vi "Stepper -- V5.vi"() -> ()   [LabVIEW 2019]
doc: "Use this template to build a producer/consumer design pattern with events to produce queue items. Use this design pattern instead of the User Interface Event Handler pattern for user interfaces when you want to execute code asynchronously in response to an event without slowing the user interface responsiveness."
uses:
  stepper motor state.ctl
  cursor range mode.ctl
  motor type.ctl
  stepper graphics action.ctl
  stepper driver action.ctl
  stepper progress monitor message.ctl
  talkto async routine action.ctl
  stepper graphics internal state.ctl
  stepper graphics internal event.ctl
  slider action.ctl
  stepper driver -- BLM.vi
  publisher action.ctl
panel:
  in  "Tab Control":enum32{"main", "init&stuff", "ignore", "calc"}(tab)
  in  "cur step":dbl(slide) scale=-5725.0..5322.0 scale format="%#.0f"
  in  "set step !":dbl(slide)=882.0 min=0.0 max=16000.0 step=1.0 scale=-5725.0..5322.0
  in  "set angle!":dbl(slide)=21.577803928668402 scale=-110.0..110.0
  in  "Stop!":bool
  in  "Go!":bool
  in  "check!":bool
  in  "stepper state":T1=enum."stopped"
  in  "XY Graph":cluster{dbl[], dbl[]}[](graph)=[{[-0.27897570766599245, -0.2006667370930823, -0.12235776652017213, -0.044048795947261965, 0.034260174625648177, 0.11256914519855832, 0.19087811577146852, 0.2691870863443786, 0.3474960569172888, 0.425805027490199, 0.5041139980631091, 0.5824229686360193, 0.6607319392089295, 0.7390409097818396, 0.8173498803547496, 0.89565885092766, 0.97396782150057, 1.0522767920734801, 1.1305857626463904, 1.2088947332193005], [-0.11032930042494946, -0.07935967223548995, -0.04839004404603046, -0.01742041585657096, 0.013549212332888541, 0.04451884052234803, 0.07548846871180753, 0.10645809690126704, 0.13742772509072654, 0.16839735328018604, 0.19936698146964552, 0.23033660965910505, 0.26130623784856455, 0.292275866038024, 0.3232454942274835, 0.3542151224169431, 0.38518475060640256, 0.41615437879586203, 0.4471240069853215, 0.478093635174781]}, {[-0.29926451263811893, -0.23626145734588336, -0.1732584020536478, -0.11025534676141222, -0.047252291469176644, 0.015750763823058955, 0.0787538191152945, 0.14175687440753004, 0.20475992969976564, 0.26776298499200124, 0.33076604028423684, 0.3937690955764723, 0.4567721508687079, 0.5197752061609435, 0.582778261453179, 0.6457813167454146, 0.7087843720376502, 0.7717874273298858, 0.8347904826221214, 0.897793537914357], [-0.020994081915366267, -0.01657427519634179, -0.01215446847731731, -0.007734661758292832, -0.0033148550392683544, 0.0011049516797561228, 0.005524758398780603, 0.00994456511780508, 0.014364371836829558, 0.018784178555854035, 0.023203985274878512, 0.02762379199390299, 0.032043598712927474, 0.03646340543195195, 0.04088321215097643, 0.045303018870000905, 0.04972282558902538, 0.05414263230804986, 0.05856243902707434, 0.06298224574609881]}, {[1.0, 0.9980267284282716, 0.9921147013144779, 0.9822872507286887, 0.9685831611286311, 0.9510565162951535, 0.9297764858882513, 0.9048270524660195, 0.8763066800438636, 0.8443279255020151, 0.8090169943749475, 0.7705132427757891, 0.7289686274214116, 0.6845471059286886, 0.6374239897486896, 0.587785252292473, 0.5358267949789965, 0.48175367410171516, 0.42577929156507266, 0.36812455268467786, 0.30901699437494745, 0.24868988716485474, 0.18738131458572452, 0.12533323356430426, 0.0627905195293133, -1.6081428723391245e-16, -0.0627905195293134, -0.12533323356430437, -0.18738131458572482, -0.24868988716485485, -0.30901699437494756, -0.368124552684678, -0.4257792915650727, -0.48175367410171543, -0.5358267949789969, -0.587785252292473, -0.6374239897486897, -0.6845471059286887, -0.7289686274214117, -0.7705132427757894, -0.8090169943749473, -0.8443279255020151, -0.8763066800438636, -0.9048270524660196, -0.9297764858882515, -0.9510565162951536, -0.9685831611286311, -0.9822872507286887, -0.9921147013144779, -0.9980267284282716, -1.0, -0.9980267284282716, -0.9921147013144779, -0.9822872507286886, -0.9685831611286311, -0.9510565162951535, -0.9297764858882512, -0.9048270524660195, -0.8763066800438635, -0.844327925502015, -0.8090169943749472, -0.770513242775789, -0.7289686274214116, -0.6845471059286886, -0.6374239897486895, -0.5877852522924732, -0.5358267949789963, -0.48175367410171527, -0.42577929156507216, -0.3681245526846778, -0.30901699437494756, -0.24868988716485443, -0.18738131458572463, -0.12533323356430373, -0.06279051952931321, -1.836909530733566e-16, 0.06279051952931372, 0.12533323356430423, 0.18738131458572513, 0.24868988716485493, 0.30901699437494723, 0.36812455268467825, 0.4257792915650726, 0.4817536741017157, 0.5358267949789968, 0.5877852522924737, 0.63742398974869, 0.6845471059286886, 0.7289686274214119, 0.7705132427757894, 0.8090169943749478, 0.8443279255020153, 0.8763066800438636, 0.9048270524660197, 0.9297764858882515, 0.9510565162951538, 0.9685831611286312, 0.9822872507286887, 0.9921147013144779, 0.9980267284282716], [0.0, 0.06279051952931337, 0.12533323356430426, 0.18738131458572463, 0.2486898871648548, 0.3090169943749474, 0.368124552684678, 0.4257792915650727, 0.4817536741017153, 0.5358267949789967, 0.5877852522924731, 0.6374239897486897, 0.6845471059286887, 0.7289686274214116, 0.7705132427757893, 0.8090169943749475, 0.8443279255020151, 0.8763066800438637, 0.9048270524660196, 0.9297764858882515, 0.9510565162951535, 0.9685831611286311, 0.9822872507286887, 0.9921147013144779, 0.9980267284282716, 1.0, 0.9980267284282716, 0.9921147013144778, 0.9822872507286886, 0.9685831611286311, 0.9510565162951535, 0.9297764858882513, 0.9048270524660195, 0.8763066800438635, 0.844327925502015, 0.8090169943749475, 0.7705132427757893, 0.7289686274214114, 0.6845471059286885, 0.6374239897486895, 0.5877852522924732, 0.5358267949789967, 0.4817536741017152, 0.4257792915650725, 0.36812455268467775, 0.3090169943749471, 0.24868988716485482, 0.18738131458572457, 0.1253332335643041, 0.06279051952931314, -3.216285744678249e-16, -0.06279051952931335, -0.12533323356430429, -0.18738131458572477, -0.24868988716485502, -0.30901699437494773, -0.3681245526846783, -0.42577929156507266, -0.4817536741017154, -0.5358267949789968, -0.5877852522924734, -0.63742398974869, -0.6845471059286887, -0.7289686274214116, -0.7705132427757894, -0.8090169943749473, -0.8443279255020153, -0.8763066800438636, -0.9048270524660198, -0.9297764858882515, -0.9510565162951535, -0.9685831611286312, -0.9822872507286887, -0.9921147013144779, -0.9980267284282716, -1.0, -0.9980267284282716, -0.9921147013144779, -0.9822872507286886, -0.9685831611286311, -0.9510565162951536, -0.9297764858882512, -0.9048270524660196, -0.8763066800438634, -0.844327925502015, -0.809016994374947, -0.770513242775789, -0.7289686274214116, -0.6845471059286883, -0.6374239897486896, -0.5877852522924726, -0.5358267949789963, -0.4817536741017153, -0.4257792915650722, -0.36812455268467786, -0.3090169943749468, -0.2486898871648545, -0.18738131458572468, -0.1253332335643038, -0.06279051952931326]}, {[0.1, 0.09980267284282716, 0.0992114701314478, 0.09822872507286887, 0.09685831611286312, 0.09510565162951537, 0.09297764858882515, 0.09048270524660196, 0.08763066800438636, 0.08443279255020152, 0.08090169943749474, 0.07705132427757892, 0.07289686274214115, 0.06845471059286887, 0.06374239897486897, 0.05877852522924731, 0.05358267949789966, 0.04817536741017152, 0.042577929156507266, 0.03681245526846779, 0.03090169943749475, 0.024868988716485477, 0.018738131458572452, 0.012533323356430426, 0.00627905195293133, -1.6081428723391246e-17, -0.0062790519529313405, -0.012533323356430436, -0.018738131458572484, -0.024868988716485487, -0.030901699437494757, -0.0368124552684678, -0.04257792915650727, -0.048175367410171546, -0.05358267949789969, -0.05877852522924731, -0.06374239897486897, -0.06845471059286888, -0.07289686274214117, -0.07705132427757895, -0.08090169943749474, -0.08443279255020152, -0.08763066800438636, -0.09048270524660197, -0.09297764858882515, -0.09510565162951537, -0.09685831611286312, -0.09822872507286888, -0.0992114701314478, -0.09980267284282716, -0.1, -0.09980267284282716, -0.0992114701314478, -0.09822872507286887, -0.09685831611286311, -0.09510565162951536, -0.09297764858882514, -0.09048270524660196, -0.08763066800438636, -0.0844327925502015, -0.08090169943749473, -0.07705132427757891, -0.07289686274214116, -0.06845471059286887, -0.06374239897486896, -0.05877852522924733, -0.05358267949789963, -0.04817536741017153, -0.04257792915650722, -0.036812455268467784, -0.03090169943749476, -0.024868988716485445, -0.018738131458572463, -0.012533323356430372, -0.0062790519529313206, -1.836909530733566e-17, 0.006279051952931373, 0.012533323356430424, 0.018738131458572515, 0.024868988716485498, 0.030901699437494726, 0.03681245526846783, 0.042577929156507266, 0.048175367410171574, 0.053582679497899674, 0.05877852522924737, 0.063742398974869, 0.06845471059286887, 0.07289686274214119, 0.07705132427757894, 0.08090169943749478, 0.08443279255020153, 0.08763066800438636, 0.09048270524660197, 0.09297764858882515, 0.09510565162951538, 0.09685831611286312, 0.09822872507286887, 0.0992114701314478, 0.09980267284282716], [0.0, 0.006279051952931338, 0.012533323356430426, 0.018738131458572466, 0.02486898871648548, 0.030901699437494743, 0.0368124552684678, 0.04257792915650727, 0.04817536741017153, 0.05358267949789967, 0.058778525229247314, 0.06374239897486898, 0.06845471059286887, 0.07289686274214116, 0.07705132427757894, 0.08090169943749476, 0.08443279255020152, 0.08763066800438638, 0.09048270524660196, 0.09297764858882515, 0.09510565162951536, 0.09685831611286312, 0.09822872507286888, 0.0992114701314478, 0.09980267284282716, 0.1, 0.09980267284282716, 0.0992114701314478, 0.09822872507286887, 0.09685831611286312, 0.09510565162951536, 0.09297764858882515, 0.09048270524660196, 0.08763066800438636, 0.0844327925502015, 0.08090169943749476, 0.07705132427757892, 0.07289686274214115, 0.06845471059286885, 0.06374239897486896, 0.05877852522924732, 0.05358267949789967, 0.048175367410171525, 0.04257792915650725, 0.03681245526846778, 0.030901699437494712, 0.024868988716485484, 0.01873813145857246, 0.01253332335643041, 0.0062790519529313145, -3.216285744678249e-17, -0.0062790519529313344, -0.012533323356430431, -0.018738131458572477, -0.0248689887164855, -0.030901699437494774, -0.03681245526846783, -0.04257792915650727, -0.04817536741017154, -0.05358267949789968, -0.05877852522924734, -0.06374239897486901, -0.06845471059286887, -0.07289686274214116, -0.07705132427757894, -0.08090169943749474, -0.08443279255020153, -0.08763066800438636, -0.09048270524660199, -0.09297764858882515, -0.09510565162951536, -0.09685831611286312, -0.09822872507286888, -0.0992114701314478, -0.09980267284282716, -0.1, -0.09980267284282716, -0.0992114701314478, -0.09822872507286887, -0.09685831611286311, -0.09510565162951537, -0.09297764858882514, -0.09048270524660196, -0.08763066800438633, -0.0844327925502015, -0.0809016994374947, -0.07705132427757891, -0.07289686274214116, -0.06845471059286884, -0.06374239897486897, -0.058778525229247265, -0.05358267949789964, -0.04817536741017153, -0.042577929156507224, -0.036812455268467784, -0.03090169943749468, -0.024868988716485452, -0.01873813145857247, -0.012533323356430379, -0.006279051952931327]}, {[-1.7, -1.7, -1.7, -1.7, -1.7, -1.7, -1.7, -1.7, -1.7, -1.7, -1.7, -1.7, -1.7, -1.7, -1.7, -1.7, -1.7, -1.7, -1.7, -1.7, -1.7, -1.6105263157894736, -1.5210526315789474, -1.431578947368421, -1.3421052631578947, -1.2526315789473683, -1.163157894736842, -1.0736842105263158, -0.9842105263157894, -0.894736842105263, -0.8052631578947368, -0.7157894736842105, -0.6263157894736842, -0.5368421052631578, -0.44736842105263164, -0.35789473684210527, -0.2684210526315789, -0.17894736842105252, -0.08947368421052615, 0.0, 0.0, 0.08947368421052632, 0.17894736842105263, 0.26842105263157895, 0.35789473684210527, 0.4473684210526316, 0.5368421052631579, 0.6263157894736842, 0.7157894736842105, 0.8052631578947369, 0.8947368421052632, 0.9842105263157894, 1.0736842105263158, 1.1631578947368422, 1.2526315789473683, 1.3421052631578947, 1.431578947368421, 1.5210526315789474, 1.6105263157894738, 1.7, 1.7, 1.7, 1.7, 1.7, 1.7, 1.7, 1.7, 1.7, 1.7, 1.7, 1.7, 1.7, 1.7, 1.7, 1.7, 1.7, 1.7, 1.7, 1.7, 1.7], [1.9, 1.7210526315789472, 1.5421052631578946, 1.3631578947368421, 1.1842105263157894, 1.0052631578947366, 0.8263157894736841, 0.6473684210526316, 0.46842105263157885, 0.2894736842105261, 0.11052631578947358, -0.06842105263157894, -0.24736842105263168, -0.4263157894736844, -0.6052631578947367, -0.7842105263157895, -0.9631578947368422, -1.142105263157895, -1.3210526315789477, -1.5, -1.5, -1.5257894736842106, -1.551578947368421, -1.5773684210526315, -1.6031578947368421, -1.6289473684210527, -1.654736842105263, -1.6805263157894736, -1.7063157894736842, -1.7321052631578948, -1.7578947368421052, -1.7836842105263158, -1.8094736842105263, -1.8352631578947367, -1.8610526315789473, -1.8868421052631579, -1.9126315789473685, -1.938421052631579, -1.9642105263157894, -1.99, -1.9900000000000002, -1.9642105263157896, -1.9384210526315793, -1.9126315789473687, -1.886842105263158, -1.8610526315789475, -1.8352631578947372, -1.8094736842105266, -1.783684210526316, -1.7578947368421054, -1.732105263157895, -1.7063157894736845, -1.6805263157894739, -1.6547368421052635, -1.628947368421053, -1.6031578947368423, -1.5773684210526318, -1.5515789473684212, -1.5257894736842108, -1.5000000000000002, -1.5, -1.3210526315789473, -1.1421052631578947, -0.9631578947368421, -0.7842105263157895, -0.6052631578947368, -0.4263157894736842, -0.24736842105263168, -0.06842105263157894, 0.1105263157894738, 0.2894736842105263, 0.46842105263157885, 0.6473684210526316, 0.8263157894736843, 1.0052631578947366, 1.1842105263157894, 1.3631578947368421, 1.5421052631578949, 1.7210526315789476, 1.9]}, {[-0.3420201433256687, -0.3492205673956828, -0.3564209914656969, -0.3636214155357109, -0.370821839605725, -0.3780222636757391, -0.3852226877457532, -0.3924231118157673, -0.3996235358857813, -0.4068239599557954, -0.4140243840258095, -0.4212248080958236, -0.4284252321658376, -0.4356256562358517, -0.4428260803058658, -0.4500265043758799, -0.45722692844589397, -0.46442735251590805, -0.47162777658592214, -0.4788282006559362], [0.9396926207859084, 0.9594756233287697, 0.9792586258716309, 0.9990416284144921, 1.0188246309573534, 1.0386076335002146, 1.0583906360430757, 1.078173638585937, 1.0979566411287982, 1.1177396436716593, 1.1375226462145207, 1.1573056487573818, 1.177088651300243, 1.1968716538431043, 1.2166546563859655, 1.2364376589288266, 1.256220661471688, 1.2760036640145493, 1.2957866665574105, 1.3155696691002716]}, {[-0.3420201433256687, -0.3492205673956828, -0.3564209914656969, -0.3636214155357109, -0.370821839605725, -0.3780222636757391, -0.3852226877457532, -0.3924231118157673, -0.3996235358857813, -0.4068239599557954, -0.4140243840258095, -0.4212248080958236, -0.4284252321658376, -0.4356256562358517, -0.4428260803058658, -0.4500265043758799, -0.45722692844589397, -0.46442735251590805, -0.47162777658592214, -0.4788282006559362], [-0.9396926207859084, -0.9594756233287697, -0.9792586258716309, -0.9990416284144921, -1.0188246309573534, -1.0386076335002146, -1.0583906360430757, -1.078173638585937, -1.0979566411287982, -1.1177396436716593, -1.1375226462145207, -1.1573056487573818, -1.177088651300243, -1.1968716538431043, -1.2166546563859655, -1.2364376589288266, -1.256220661471688, -1.2760036640145493, -1.2957866665574105, -1.3155696691002716]}, {[-0.4788282006559362, -0.42797342694834783, -0.37648774886137176, -0.3244470648918203, -0.27192809170796073, -0.2190082510563231, -0.16576555562910145, -0.11227849406040255, -0.058625915220879475, -0.004886911981313146, 0.04885929538350151, 0.10253347597868427, 0.15605650508885563, 0.2093494808211934, 0.2623338404200143, 0.31493147608141087, 0.36706485009721057, 0.41865710915852133, 0.4696321976503571, 0.5199149697703286, 0.5694313003061202, 0.6181081939084433, 0.6658738926983852, 0.7126579820505197, 0.7583914943958358, 0.8030070108914645, 0.8464387608073247, 0.8886227184831744, 0.9294966977131381, 0.9690004434185695, 1.0070757204741114, 1.043666399556007, 1.0787185398861048, 1.1121804687495853, 1.1440028576691799, 1.1741387951235935, 1.20254385570293, 1.2291761655991726, 1.2539964643351778, 1.276968162641182, 1.2980573963935023, 1.3172330765359155, 1.3344669349101257, 1.349733565927754, 1.3630104640224243, 1.3742780568267294, 1.383519734025174, 1.390721871840555, 1.3958738531176882, 1.3989680829748696, 1.4, 1.3989680829748696, 1.3958738531176882, 1.390721871840555, 1.383519734025174, 1.3742780568267294, 1.3630104640224243, 1.3497335659277543, 1.3344669349101257, 1.3172330765359157, 1.2980573963935025, 1.2769681626411822, 1.253996464335178, 1.2291761655991726, 1.2025438557029302, 1.1741387951235938, 1.1440028576691799, 1.1121804687495855, 1.0787185398861048, 1.0436663995560072, 1.0070757204741119, 0.9690004434185695, 0.9294966977131384, 0.888622718483175, 0.8464387608073248, 0.8030070108914648, 0.7583914943958362, 0.7126579820505199, 0.6658738926983856, 0.6181081939084433, 0.5694313003061205, 0.5199149697703291, 0.4696321976503571, 0.41865710915852167, 0.36706485009721057, 0.3149314760814112, 0.2623338404200149, 0.2093494808211934, 0.15605650508885596, 0.1025334759786849, 0.04885929538350151, -0.004886911981312835, -0.05862591522087885, -0.11227849406040225, -0.16576555562910084, -0.2190082510563231, -0.27192809170796045, -0.3244470648918197, -0.37648774886137176, -0.4279734269483475], [-1.3155696691002716, -1.332981149838994, -1.3484275935167214, -1.361886229493155, -1.373337217488868, -1.3827636768331928, -1.3901517113491517, -1.395490429838746, -1.3987719621384016, -1.3999914707209065, -1.3991471578267338, -1.3962402681142412, -1.391275086824835, -1.3842589334658082, -1.3752021510201642, -1.3641180906993293, -1.351023092261236, -1.3359364599227874, -1.3188804339022153, -1.299880157633279, -1.2789636406996412, -1.2561617175440598, -1.2315080020132632, -1.205038837805521, -1.176793244893958, -1.1468128620045883, -1.1151418852338748, -1.0818270028962915, -1.0469173266979446, -1.010464319337707, -0.9725217186425963, -0.9331454583492336, -0.8923935856481656, -0.8503261756126013, -0.8070052426377105, -0.762494649021038, -0.7168600108188002, -0.6701686011168495, -0.6224892508588987, -0.573892247378202, -0.5244492307822769, -0.47423308834340794, -0.42331784705062225, -0.3717785644815325, -0.31969121815491813, -0.2671325935271628, -0.21418017079765359, -0.16091201069001346, -0.10740663937754624, -0.05374293272252798, 0.0, 0.05374293272252768, 0.10740663937754594, 0.16091201069001315, 0.21418017079765295, 0.2671325935271628, 0.31969121815491786, 0.3717785644815319, 0.42331784705062225, 0.47423308834340766, 0.5244492307822763, 0.5738922473782017, 0.6224892508588982, 0.6701686011168495, 0.7168600108187999, 0.7624946490210375, 0.8070052426377105, 0.850326175612601, 0.8923935856481656, 0.9331454583492333, 0.9725217186425958, 1.010464319337707, 1.0469173266979444, 1.081827002896291, 1.1151418852338746, 1.1468128620045883, 1.1767932448939575, 1.205038837805521, 1.2315080020132627, 1.2561617175440598, 1.278963640699641, 1.2998801576332786, 1.3188804339022153, 1.3359364599227874, 1.351023092261236, 1.364118090699329, 1.375202151020164, 1.3842589334658082, 1.391275086824835, 1.3962402681142412, 1.3991471578267338, 1.3999914707209065, 1.3987719621384016, 1.395490429838746, 1.3901517113491517, 1.3827636768331928, 1.3733372174888683, 1.3618862294931553, 1.3484275935167214, 1.3329811498389943]}]
  in  "motor selector":T2=enum."BLM"
  in  "Instrument Address":refnum<visa-resource-name>="ASRL21::INSTR"
  in  "set speed!":bool
  in  "speed":dbl=0.4 format="%_2f"
  in  "sync to":bool
  in  "syncto":dbl format="%_2f"
  in  "cursor mode":T3
  in  "response message":cluster{"step (fdeg)":dbl}={"step (fdeg)"=310.3875004849805}
  out "progress monitor VI":refnum<vi>
  out "cur angle":dbl(slide)=4.0128541685525505 scale=-110.0..110.0 scale format="%#.0f"
  in  "angle aux":dbl(slide)=110.0 scale=-90.0..90.0 scale format="%#.0f"
  in  "step aux":dbl(slide)=5322.333333333334 scale=-4721.0..4318.0 scale format="%#.0f"
  in  "dir":u16(ring)
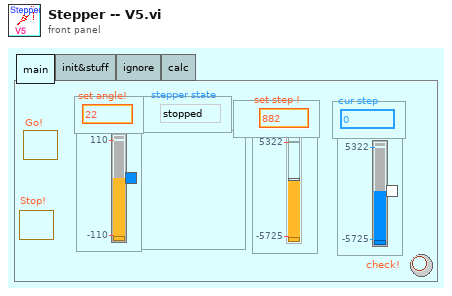
[diagram p1: front panel]
types:
  T1 = typedef "stepper motor state.ctl" = enum16{"moving", "stopped"}
  T2 = typedef "motor type.ctl" = enum16{"IMS", "arduino C&A", "BLM", "--"}
  T3 = typedef "cursor range mode.ctl" = enum16{"change angle", "lock", "extend"}
  T4 = typedef "stepper graphics action.ctl" = enum16{"--update circle", "set step slider moves", "cursor moves", "current step changed", "init", "void", "--draw current line", "--draw set line", "--move current step slider", "--move set step slider", "--draw limit lines", "check", "--move set angle slider", "--move current angle slider", "set angle slider moves", "--move center cursor", "set set step", "set current step", "read", "--move limit-cursors", "cursor release", "current step moves"}
  T5 = typedef "stepper driver action.ctl" = enum16{"go", "void", "stop", "check", "init", "sync", "set", "set speed", "--check status", "--check value", "--handshake"}
  T6 = typedef "stepper graphics internal event.ctl" = enum16{"set slider moves", "update scale", "exit", "current positon changed", "stop", "go", "set speed", "set to zero", "sync", "check"}
  T7 = typedef "stepper graphics internal state.ctl" = cluster{"set pos slider":refnum<vi>, "cur angle slider":refnum<vi>, "XY Graph":refnum<vi>, "set angle":dbl, "current angle":dbl, "set angle slider":refnum<vi>, "current pos... slider":refnum<vi>, "current pos":dbl, "set pos":dbl}
  T8 = typedef "talkto async routine action.ctl" = enum16{"stop", "check"}
  T9 = typedef "stepper progress monitor message.ctl" = cluster{"current position":dbl, "stepper motor state OUT":T1}
  T10 = typedef "publisher action.ctl" = enum16{"set", "get", "init", "check"}
  T11 = typedef "slider action.ctl" = enum16{"check", "copy range -- keep value", "set from value", "set from ratio", "set from slider", "read using other slider", "set lower limit", "set upper limit", "set lower from slider", "set upper from slider", "copy range -- keep ratio", "set using other slider -- no check"}
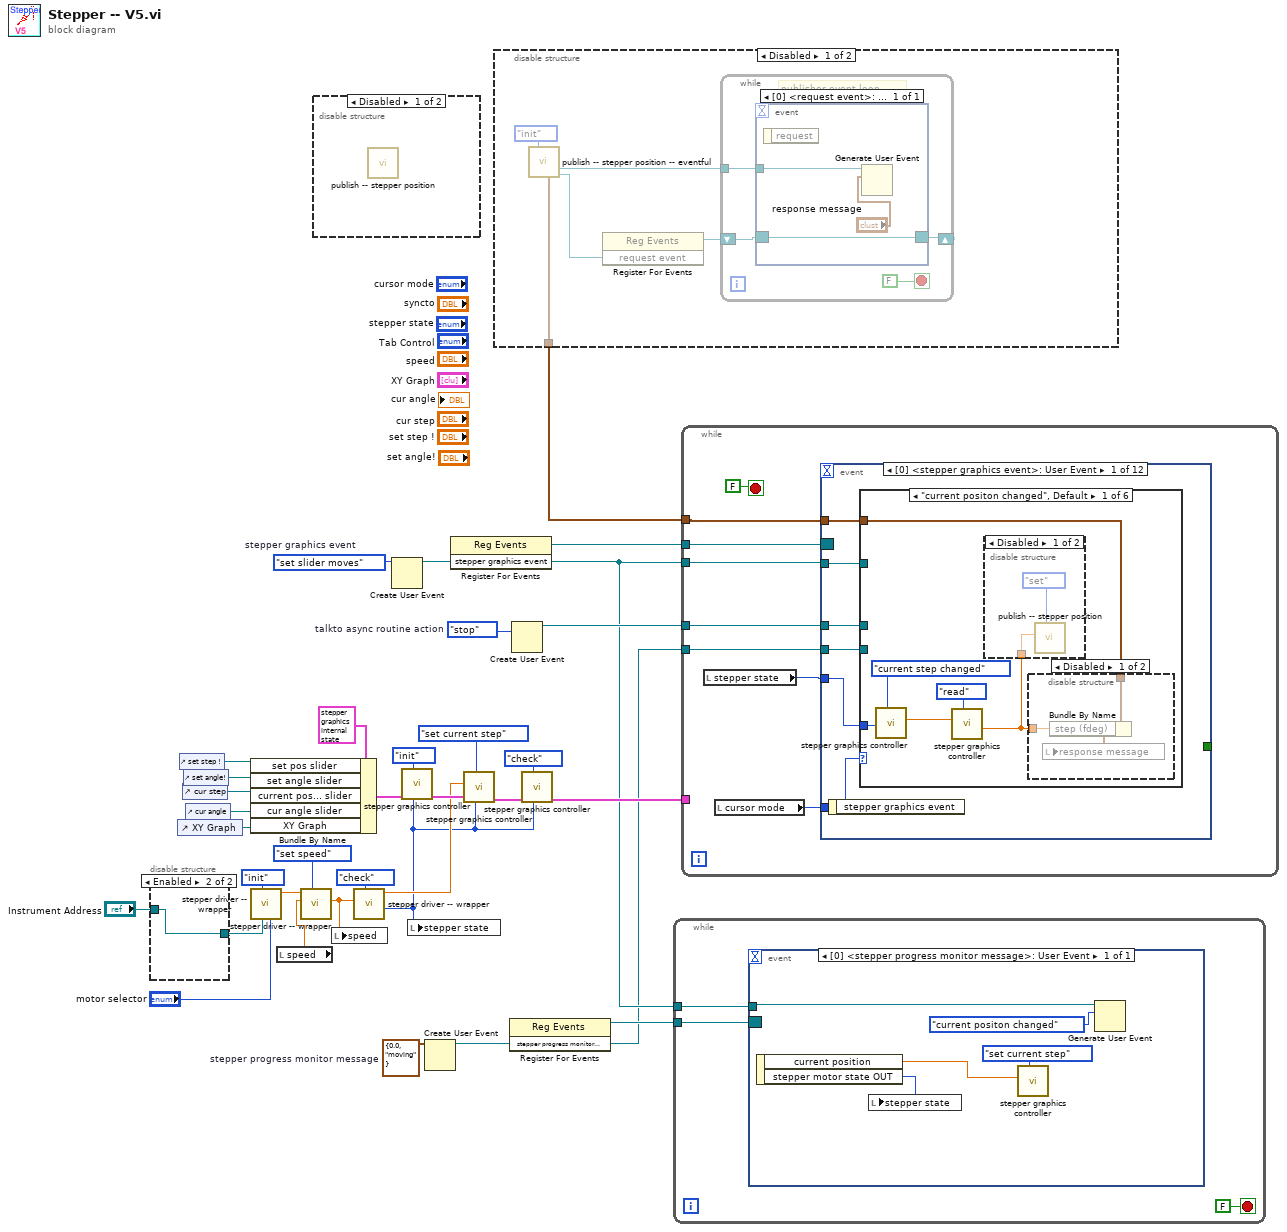
[diagram p0: block diagram]
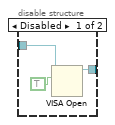
[diagram p2: hidden frame]
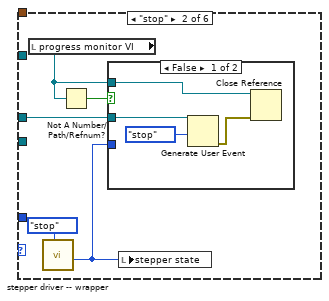
[diagram p7: hidden frame]
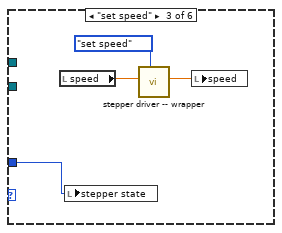
[diagram p9: hidden frame]
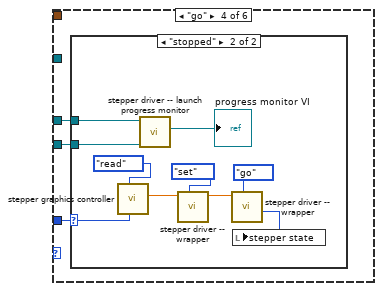
[diagram p10: hidden frame]
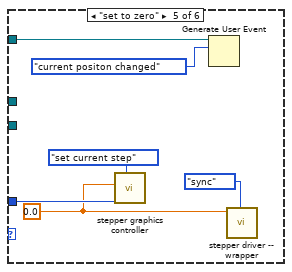
[diagram p12: hidden frame]
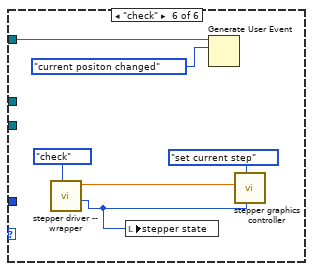
[diagram p13: hidden frame]
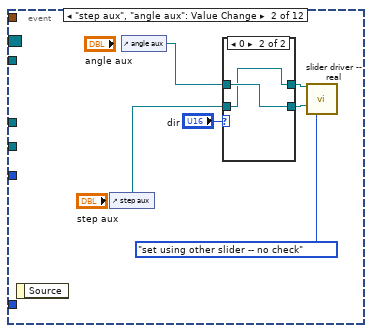
[diagram p14: hidden frame]
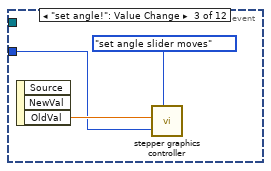
[diagram p16: hidden frame]
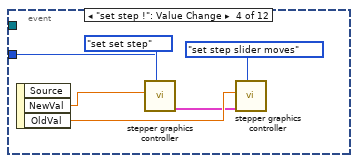
[diagram p17: hidden frame]
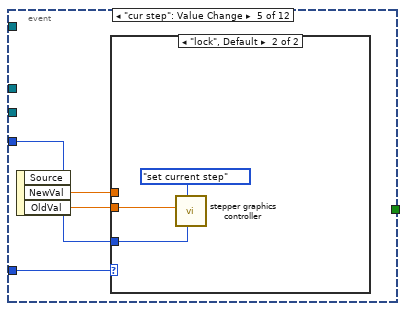
[diagram p18: hidden frame]
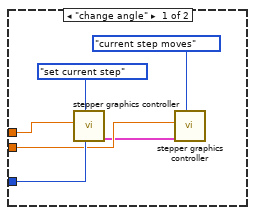
[diagram p19: hidden frame]
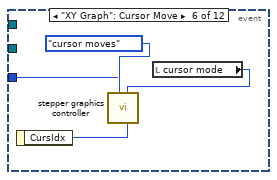
[diagram p20: hidden frame]
diagram:
  w19 = stepper_graphics_internal_event."set slider moves"  # stepper graphics event
  w28 = talkto_async_routine_action."stop"  # talkto async routine action
  w29 = T9 {"current position"=0.0, "stepper motor state OUT"=enum."moving"}  # stepper progress monitor message
  n1 = disable-structure shown="Enabled" {
    disable-tunnel: "Instrument Address" -> [w35 w37]
    disable-tunnel: [w34 w37] -> w18
    frame Disabled {
      n2 = VISA Open(duplicate session (F)=TRUE, VISA resource name=w35) -> (VISA resource name=w34:refnum<visa-resource-name>)  [unwired: 3 in, 1 out]
    }
    frame Enabled {
    }
  }
  n3 = control-ref of="XY Graph"() -> (w22:refnum<vi>)
  n4 = control-ref of="set step !"() -> (w26:refnum<vi>)
  n5 = control-ref of="cur step"() -> (w24:refnum<vi>)
  n6 = control-ref of="set angle!"() -> (w25:refnum<vi>)
  n7 = control-ref of="cur angle"() -> (w23:refnum<vi>)
  n8 = Bundle By Name(cluster=T7 {"set pos slider"=refnum, "cur angle slider"=refnum, "XY Graph"=refnum, "set angle"=0.0, "current angle"=0.0, "set angle slider"=refnum, "current pos... slider"=refnum, "current pos"=0.0, "set pos"=0.0} ("stepper graphics internal state"), "set pos slider"=w26, "set angle slider"=w25, "current pos... slider"=w24, "cur angle slider"=w23, "XY Graph"=w22) -> (w20:T7)
  n9 = call "stepper driver -- wrapper.vi"("motor selector"="motor selector", "Instrument Address"=w18, "stepper driver action"=stepper_driver_action."init") -> ("number OUT"=w16:dbl)  [unwired: 6 in, 2 out]
  n10 = local read "speed"() -> (w17:dbl)
  n11 = call "stepper driver -- wrapper.vi"("stepper driver action"=stepper_driver_action."set speed", "speed IN"=w17, "number IN"=w16) -> ("speed OUT"=w10:dbl)  [unwired: 6 in, 2 out]
  n12 = disable-structure shown="Disabled" {
    frame Disabled {
      n13 = call "publish -- stepper position.vi"() -> ()  [unwired: 11 in, 1 out]
    }
    frame Enabled {
    }
  }
  n14 = local write "speed"(w10) -> ()
  n15 = call "stepper driver -- wrapper.vi"("stepper driver action"=stepper_driver_action."check", "speed IN"=w10) -> ("stepper motor state OUT"=w5:T1, "number OUT"=w11:dbl)  [unwired: 7 in, 1 out]
  n16 = Create User Event(user event datatype=w19) -> (user event=w2:refnum<user-event>)  [unwired: 1 in, 1 out]
  n17 = call "stepper graphics controller.vi"("stepper motor state"=w5, "stepper graphics action"=stepper_graphics_action."init", "stepper graphics internal state"=w20) -> ("stepper graphics internal state OUT"=w12:T7)  [unwired: 6 in, 2 out]
  n18 = local write "stepper state"(w5) -> ()
  n19 = Create User Event(user event datatype=w29) -> (user event=w1:refnum<user-event>)  [unwired: 1 in, 1 out]
  n20 = register-events(w2) -> (reference out=w32:refnum<event-registration>)  [unwired: 2 in, 1 out]
  n21 = call "stepper graphics controller.vi"("stepper motor state"=w5, "stepper graphics action"=stepper_graphics_action."set current step", "stepper graphics internal state"=w12, "value"=w11) -> ("stepper graphics internal state OUT"=w8:T7)  [unwired: 5 in, 2 out]
  n22 = disable-structure shown="Disabled" {
    disable-tunnel: [w38 _] -> w15
    frame Disabled {
      n23 = call "publish -- stepper position -- eventful.vi"("publisher action"=publisher_action."init") -> ("response event"=w39:refnum<user-event>, "response type"=w38:cluster{"step (fdeg)":dbl}, "request event"=w40:refnum<user-event>)  [unwired: 11 in, 1 out]
      n24 = register-events(w40) -> (reference out=w41:refnum<event-registration>)  [unwired: 2 in, 1 out]
      n25 = while {
        shift-right: [w45] -> _
        shift-left: w41 -> [w44]
        tunnel: w39 -> [w43]
        stop <- FALSE stop-if-true
        # "publisher event loop"
        n26 = event shown="[0] <request event>: User Event" {
          selector: w44 -> [w49]
          dyn-events: [w49] -> w45
          timeout: _ -> [_]
          tunnel: w43 -> [w48]
          event User Event {
            n27 = event-data() -> ()  [unwired: 1 in, 1 out]
            n28 = Generate User Event(user event=w48, event data cluster="response message") -> ()  [unwired: 2 in, 2 out]
          }
        }
      }
    }
    frame Enabled {
    }
  }
  n29 = register-events(w1) -> (reference out=w4:refnum<event-registration>)  [unwired: 2 in, 1 out]
  n30 = Create User Event(user event datatype=w28) -> (user event=w3:refnum<user-event>)  [unwired: 1 in, 1 out]
  n31 = call "stepper graphics controller.vi"("stepper motor state"=w5, "stepper graphics action"=stepper_graphics_action."check", "stepper graphics internal state"=w8) -> ("stepper graphics internal state OUT"=w7:T7)  [unwired: 6 in, 2 out]
  n32 = while {
    tunnel: w4 -> [w52]
    tunnel: w2 -> [w51]
    stop <- FALSE stop-if-true
    n33 = event shown="[0] <stepper progress monitor message>: User Event" {
      selector: w52 -> [_]
      dyn-events: _ -> [_]
      timeout: _ -> [_]
      tunnel: w51 -> [w57]
      event User Event {
        n34 = event-data() -> ("current position"=w53:dbl, "stepper motor state OUT"=w54:T1)  [unwired: 1 in]
        n35 = local write "stepper state"(w54) -> ()
        n36 = call "stepper graphics controller.vi"("stepper graphics action"=stepper_graphics_action."set current step", "value"=w53) -> ()  [unwired: 7 in, 3 out]
        n37 = Generate User Event(user event=w57, event data cluster=stepper_graphics_internal_event."current positon changed" ("event data")) -> ()  [unwired: 2 in, 2 out]
      }
    }
  }
  n38 = while {
    tunnel: w32 -> [w65]
    tunnel: w2 -> [w64]
    tunnel: w1 -> [w62]
    tunnel: w3 -> [w61]
    tunnel: w15 -> [w59]
    tunnel: w7 -> [_]
    stop <- FALSE stop-if-true
    n39 = local read "stepper state"() -> (w63:T1)
    n40 = local read "cursor mode"() -> (w58:T3)
    n41 = event shown="[0] <stepper graphics event>: User Event" {
      selector: w65 -> [_ _ _ _ _ _ _ _ _ _ _ _]
      dyn-events: _ -> [_ _ _ _ _ _ _ _ _ _ _ _]
      timeout: _ -> [_ _ _ _ _ _ _ _ _ _ _ _]
      tunnel: w64 -> [w69 _ _ _ _ _ _ w161 w165 w168 w171 w174]
      tunnel: w63 -> [w70 _ w131 w138 w143 w155 w158 _ _ _ _ _]
      tunnel: [_ _ _ _ _ _ _ "Stop!" "set speed!" "Go!" "check!" "sync to"] -> _
      tunnel: w62 -> [w68 _ _ _ _ _ _ _ _ _ _ _]
      tunnel: w61 -> [w67 _ _ _ _ _ _ _ _ _ _ _]
      tunnel: w59 -> [w66 _ _ _ _ _ _ _ _ _ _ _]
      tunnel: w58 -> [_ _ _ _ w140 _ _ _ _ _ _ _]
      event User Event {
        n42 = event-data() -> ("stepper graphics event"=w71:T6)  [unwired: 1 in]
        n43 = case shown="\"current positon changed\", Default" w71 {
          tunnel: w70 -> [w76 _ w92 w97 w113 _]
          tunnel: w69 -> [_ _ _ _ w111 w118]
          tunnel: w68 -> [_ _ _ w98 _ _]
          tunnel: w67 -> [_ w84 _ w96 _ _]
          tunnel: w66 -> [w73 _ _ _ _ _]
          frame "current positon changed", Default {
            n44 = call "stepper graphics controller.vi"("stepper motor state"=w76, "stepper graphics action"=stepper_graphics_action."current step changed") -> ("set pos"=w74:dbl)  [unwired: 7 in, 2 out]
            n45 = call "stepper graphics controller.vi"("stepper graphics action"=stepper_graphics_action."read", "value"=w74) -> ("current pos"=w72:dbl)  [unwired: 7 in, 2 out]
            n46 = disable-structure shown="Disabled" {
              disable-tunnel: w72 -> [w79 _]
              frame Disabled {
                n47 = call "publish -- stepper position.vi"("publisher action"=publisher_action."set", "stepper pos IN"=w79) -> ()  [unwired: 9 in, 1 out]
              }
              frame Enabled {
              }
            }
            n48 = disable-structure shown="Disabled" {
              disable-tunnel: w72 -> [w82 _]
              disable-tunnel: w73 -> [w80 _]
              frame Disabled {
                n49 = Bundle By Name(cluster=w80, "step (fdeg)"=w82) -> (w81:cluster{"step (fdeg)":dbl})
                n50 = local write "response message"(w81) -> ()
              }
              frame Enabled {
              }
            }
          }
          frame "stop" {
            n51 = local read "progress monitor VI"() -> (w86:refnum<vi>)
            n52 = call "stepper driver -- wrapper.vi"("stepper driver action"=stepper_driver_action."stop") -> ("stepper motor state OUT"=w83:T1)  [unwired: 8 in, 2 out]
            n53 = Not A Number/Path/Refnum?(number/path/refnum=w86) -> (NaN/Path/Refnum?=w85:bool)
            n54 = case shown="False" w85 {
              tunnel: w86 -> [w91 _]
              tunnel: w84 -> [w90 _]
              tunnel: w83 -> [_ _]
              frame False {
                n55 = Generate User Event(user event=w90, event data cluster=talkto_async_routine_action."stop" ("event data")) -> (error out=w88:errorcluster)  [unwired: 2 in, 1 out]
                n56 = Close Reference(reference=w91, error in (no error)=w88) -> ()  [unwired: 1 out]
              }
              frame True {
              }
            }
            n57 = local write "stepper state"(w83) -> ()
          }
          frame "set speed" {
            n58 = local read "speed"() -> (w94:dbl)
            n59 = local write "stepper state"(w92) -> ()
            n60 = call "stepper driver -- wrapper.vi"("stepper driver action"=stepper_driver_action."set speed", "speed IN"=w94) -> ("speed OUT"=w93:dbl)  [unwired: 7 in, 2 out]
            n61 = local write "speed"(w93) -> ()
          }
          frame "go" {
            n62 = case shown="\"stopped\"" w97 {
              selector: w97 -> [_ w100]
              tunnel: w98 -> [_ w106]
              tunnel: w96 -> [_ w105]
              frame "moving", Default {
              }
              frame "stopped" {
                n63 = call "stepper graphics controller.vi"("stepper motor state"=w100, "stepper graphics action"=stepper_graphics_action."read") -> ("set pos"=w103:dbl)  [unwired: 7 in, 2 out]
                n64 = call "stepper driver -- launch progress monitor.vi"("talkback  user event"=w106, "talkto user event"=w105) -> ("reference out"=→"progress monitor VI":refnum<vi>)  [unwired: 9 in]
                n65 = call "stepper driver -- wrapper.vi"("stepper driver action"=stepper_driver_action."set", "number IN"=w103) -> ("number OUT"=w102:dbl)  [unwired: 7 in, 2 out]
                n66 = call "stepper driver -- wrapper.vi"("stepper driver action"=stepper_driver_action."go", "number IN"=w102) -> ("stepper motor state OUT"=w99:T1)  [unwired: 7 in, 2 out]
                n67 = local write "stepper state"(w99) -> ()
              }
            }
          }
          frame "set to zero" {
            w109 = 0.0 ("value")
            n68 = call "stepper graphics controller.vi"("stepper motor state"=w113, "stepper graphics action"=stepper_graphics_action."set current step", "value"=w109) -> ()  [unwired: 6 in, 3 out]
            n69 = Generate User Event(user event=w111, event data cluster=stepper_graphics_internal_event."current positon changed" ("event data")) -> ()  [unwired: 2 in, 2 out]
            n70 = call "stepper driver -- wrapper.vi"("stepper driver action"=stepper_driver_action."sync", "number IN"=w109) -> ()  [unwired: 7 in, 3 out]
          }
          frame "check" {
            n71 = call "stepper driver -- wrapper.vi"("stepper driver action"=stepper_driver_action."check") -> ("stepper motor state OUT"=w115:T1, "number OUT"=w117:dbl)  [unwired: 8 in, 1 out]
            n72 = local write "stepper state"(w115) -> ()
            n73 = Generate User Event(user event=w118, event data cluster=stepper_graphics_internal_event."current positon changed" ("event data")) -> ()  [unwired: 2 in, 2 out]
            n74 = call "stepper graphics controller.vi"("stepper motor state"=w115, "stepper graphics action"=stepper_graphics_action."set current step", "value"=w117) -> ()  [unwired: 6 in, 3 out]
          }
        }
      }
      event "step aux", "angle aux": Value Change {
        n75 = event-data() -> ()  [unwired: 1 in, 1 out]
        n76 = control-ref of="step aux"() -> (w122:refnum<vi>)
        n77 = control-ref of="angle aux"() -> (w124:refnum<vi>)
        n78 = case shown="0" "dir" {
          tunnel: [w128 w129] -> w125
          tunnel: w124 -> [w128 w130]
          tunnel: [w127 w130] -> w123
          tunnel: w122 -> [w127 w129]
          frame 1, Default {
          }
          frame 0 {
          }
        }
        n79 = call "slider driver -- real.vi"("slider in"=w125, "slider action"=slider_action."set using other slider -- no check", "slider from"=w123) -> ()  [unwired: 8 in, 5 out]
      }
      event "set angle!": Value Change {
        n80 = event-data() -> ("OldVal"=w133:dbl)  [unwired: 1 in, 2 out]
        n81 = call "stepper graphics controller.vi"("stepper motor state"=w131, "stepper graphics action"=stepper_graphics_action."set angle slider moves", "value"=w133) -> ()  [unwired: 6 in, 3 out]
      }
      event "set step !": Value Change {
        n82 = event-data() -> ("NewVal"=w136:dbl, "OldVal"=w135:dbl)  [unwired: 1 in, 1 out]
        n83 = call "stepper graphics controller.vi"("stepper motor state"=w138, "stepper graphics action"=stepper_graphics_action."set set step", "value"=w136) -> ("stepper graphics internal state OUT"=w134:T7)  [unwired: 6 in, 2 out]
        n84 = call "stepper graphics controller.vi"("stepper graphics action"=stepper_graphics_action."set step slider moves", "stepper graphics internal state"=w134, "value"=w135) -> ()  [unwired: 6 in, 3 out]
      }
      event "cur step": Value Change {
        n85 = event-data() -> ("NewVal"=w142:dbl, "OldVal"=w141:dbl)  [unwired: 1 in, 1 out]
        n86 = case shown="\"lock\", Default" w140 {
          tunnel: w143 -> [w148 w151]
          tunnel: w142 -> [w146 _]
          tunnel: w141 -> [w145 w150]
          frame "change angle" {
            n87 = call "stepper graphics controller.vi"("stepper motor state"=w148, "stepper graphics action"=stepper_graphics_action."set current step", "value"=w146) -> ("stepper graphics internal state OUT"=w144:T7)  [unwired: 6 in, 2 out]
            n88 = call "stepper graphics controller.vi"("stepper graphics action"=stepper_graphics_action."current step moves", "stepper graphics internal state"=w144, "value"=w145) -> ()  [unwired: 6 in, 3 out]
          }
          frame "lock", Default {
            n89 = call "stepper graphics controller.vi"("stepper motor state"=w151, "stepper graphics action"=stepper_graphics_action."set current step", "value"=w150) -> ()  [unwired: 6 in, 3 out]
          }
        }
      }
      event "XY Graph": Cursor Move {
        n90 = event-data() -> ("CursIdx"=w154:i32)  [unwired: 1 in]
        n91 = local read "cursor mode"() -> (w153:T3)
        n92 = call "stepper graphics controller.vi"("cursor index"=w154, "cursor range mode"=w153, "stepper motor state"=w155, "stepper graphics action"=stepper_graphics_action."cursor moves") -> ()  [unwired: 5 in, 3 out]
      }
      event "XY Graph": Cursor Release {
        n93 = event-data() -> ("CursIdx"=w157:i32)  [unwired: 1 in]
        n94 = call "stepper graphics controller.vi"("cursor index"=w157, "stepper motor state"=w158, "stepper graphics action"=stepper_graphics_action."cursor release") -> ()  [unwired: 6 in, 3 out]
      }
      event "Stop!": Value Change {
        n95 = event-data() -> ()  [unwired: 1 in, 1 out]
        n96 = Generate User Event(user event=w161, event data cluster=stepper_graphics_internal_event."stop" ("event data")) -> ()  [unwired: 2 in, 2 out]
      }
      event "set speed!": Value Change {
        n97 = event-data() -> ()  [unwired: 1 in, 1 out]
        n98 = Generate User Event(user event=w165, event data cluster=stepper_graphics_internal_event."set speed" ("event data")) -> ()  [unwired: 2 in, 2 out]
      }
      event "Go!": Value Change {
        n99 = event-data() -> ()  [unwired: 1 in, 1 out]
        n100 = Generate User Event(user event=w168, event data cluster=stepper_graphics_internal_event."go" ("event data")) -> ()  [unwired: 2 in, 2 out]
      }
      event "check!": Value Change {
        n101 = event-data() -> ()  [unwired: 1 in, 1 out]
        n102 = Generate User Event(user event=w171, event data cluster=stepper_graphics_internal_event."check" ("event data")) -> ()  [unwired: 2 in, 2 out]
      }
      event "sync to": Value Change {
        n103 = event-data() -> ()  [unwired: 1 in, 1 out]
        n104 = Generate User Event(user event=w174, event data cluster=stepper_graphics_internal_event."set to zero" ("event data")) -> ()  [unwired: 2 in, 2 out]
      }
    }
  }
